vi "StopGetPic.vi"() -> ()   [LabVIEW 2013]
panel:
  in  "Stop":bool
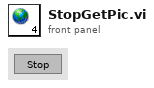
[diagram p1: front panel]
diagram:
